vi "correlation coefficient.vi"(2 "X Values":dbl[](array[numeric]) format="%.2f", 3 "Y Values":dbl[](array[numeric]) format="%.2f") -> (1 "r":dbl format="%.6f")   [LabVIEW 2015]
panel:
  # "Correlation Coefficient"
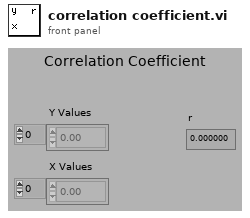
[diagram p1: front panel]
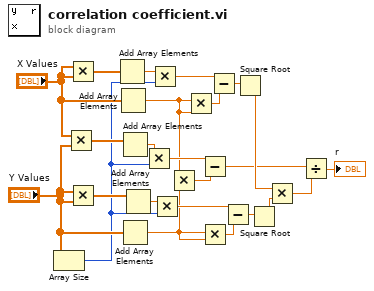
[diagram p0: block diagram]
diagram:
  n1 = Array Size(array="Y Values") -> (size(s)=w16:i32)
  n2 = Multiply(x="X Values", y="Y Values") -> (x*y=w22:dbl[])
  n3 = Multiply(x="X Values", y="X Values") -> (x*y=w24:dbl[])
  n4 = Multiply(x="Y Values", y="Y Values") -> (x*y=w20:dbl[])
  n5 = Add Array Elements(numeric array=w24) -> (sum=w15:dbl)
  n6 = Add Array Elements(numeric array="X Values") -> (sum=w13:dbl)
  n7 = Add Array Elements(numeric array=w22) -> (sum=w19:dbl)
  n8 = Add Array Elements(numeric array="Y Values") -> (sum=w7:dbl)
  n9 = Add Array Elements(numeric array=w20) -> (sum=w14:dbl)
  n10 = Multiply(x=w19, y=w16) -> (x*y=w18:dbl)
  n11 = Multiply(x=w15, y=w16) -> (x*y=w12:dbl)
  n12 = Multiply(x=w14, y=w16) -> (x*y=w8:dbl)
  n13 = Multiply(x=w13, y=w7) -> (x*y=w17:dbl)
  n14 = Multiply(x=w13, y=w13) -> (x*y=w11:dbl)
  n15 = Subtract(x=w18, y=w17) -> (x-y=w3:dbl)
  n16 = Multiply(x=w7, y=w7) -> (x*y=w9:dbl)
  n17 = Subtract(x=w12, y=w11) -> (x-y=w10:dbl)
  n18 = Subtract(x=w8, y=w9) -> (x-y=w6:dbl)
  n19 = Square Root(x=w10) -> (sqrt(x)=w4:dbl)
  n20 = Square Root(x=w6) -> (sqrt(x)=w5:dbl)
  n21 = Multiply(x=w4, y=w5) -> (x*y=w2:dbl)
  n22 = Divide(x=w3, y=w2) -> (x/y=→"r":dbl)
